vi "Write Default Object Cluster.vi"(8 "error in (no error)":errorcluster, 10 "Default":T1, 11 "ObjectSettings in":refnum<class "ObjectSettings.lvclass">) -> (0 "error out":errorcluster, 3 "ObjectSettings out":refnum<class "ObjectSettings.lvclass">)   [LabVIEW 2019, in "ObjectSettings.lvclass"]
uses:
  ObjectSettings.lvclass
  <vilib>/JDP Science/JSONtext/JSONtext.lvlib
  Typedefs/DefaultCluster.ctl
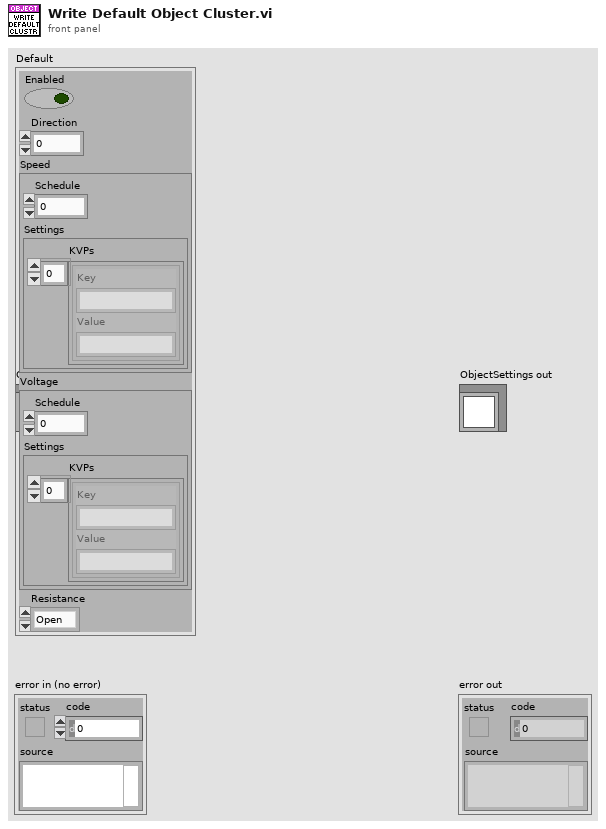
[diagram p1: front panel]
types:
  T1 = typedef "ObjectSettings.lvclass/DefaultCluster.ctl" = cluster{"Enabled":bool, "Direction":u16, "Speed":cluster{"Schedule":u16, "Settings":cluster{"KVPs":cluster{"Key":string, "Value":string}[]}}, "Voltage":cluster{"Schedule":u16, "Settings":cluster{"KVPs":cluster{"Key":string, "Value":string}[]}}, "Resistance":enum16{"Open", "Discharge Tip", "0 ohm", "100 kohm", "10 Mohm", "1 Gohm"}}
  T2 = enum16{"Open", "Discharge Tip", "0 ohm", "100 kohm", "10 Mohm", "1 Gohm"}
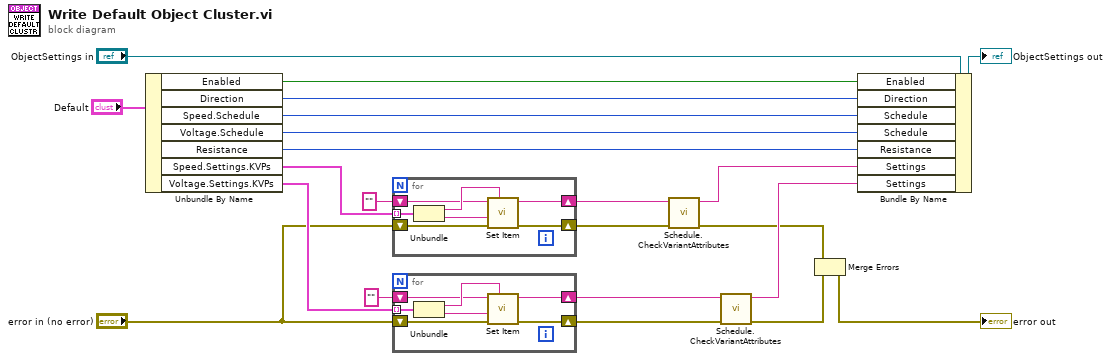
[diagram p0: block diagram]
diagram:
  n1 = Unbundle By Name("Default") -> ("Enabled"=w20:bool, "Direction"=w19:u16, "Speed.Schedule"=w15:u16, "Voltage.Schedule"=w16:u16, "Resistance"=w17:T2, "Speed.Settings.KVPs"=w1:cluster{"Key":string, "Value":string}[], "Voltage.Settings.KVPs"=w14:cluster{"Key":string, "Value":string}[])
  n2 = for {
    tunnel: w1 -> [w29] mode=indexing
    shift-right: [w23] -> w5
    shift-left: "error in (no error)" -> [w24]
    shift-right: [w25] -> w2
    shift-left: "" -> [w26]
    n3 = Unbundle(w29) -> ("Key"=w28:string, "Value"=w27:string)
    n4 = call <vilib>:"Set Item.vi"("$Path or Item Name"=w28, "error in (no error)"=w24, "JSON to Insert"=w27, "JSON"=w26) -> ("error out"=w23:errorcluster, "<JSON>"=w25:string)  [unwired: 4 in, 1 out]
  }
  n5 = for {
    tunnel: w14 -> [w36] mode=indexing
    shift-right: [w30] -> w11
    shift-left: "error in (no error)" -> [w31]
    shift-right: [w32] -> w6
    shift-left: "" -> [w33]
    n6 = Unbundle(w36) -> ("Key"=w35:string, "Value"=w34:string)
    n7 = call <vilib>:"Set Item.vi"("$Path or Item Name"=w35, "error in (no error)"=w31, "JSON to Insert"=w34, "JSON"=w33) -> ("error out"=w30:errorcluster, "<JSON>"=w32:string)  [unwired: 4 in, 1 out]
  }
  n8 = call "Schedule.CheckVariantAttributes.vi"("error in (no error)"=w5, "Schedule <JSON> In"=w2) -> ("error out"=w10:errorcluster, "Schedule <JSON> Out"=w13:string)  [unwired: 8 in]
  n9 = call "Schedule.CheckVariantAttributes.vi"("error in (no error)"=w11, "Schedule <JSON> In"=w6) -> ("error out"=w9:errorcluster, "Schedule <JSON> Out"=w12:string)  [unwired: 8 in]
  n10 = Merge Errors(w10, w9) -> (→"error out":errorcluster)
  n11 = Bundle By Name(cluster="ObjectSettings in", "Enabled"=w20, "Direction"=w19, "Schedule"=w15, "Schedule"=w16, "Resistance"=w17, "Settings"=w13, "Settings"=w12) -> (→"ObjectSettings out":refnum<class "ObjectSettings.lvclass">)
